vi "active_tracks_functional_global.vi"(4 "StimulusObjectInput":refnum<class "StimulusObject.lvclass">, 6 "Camera Frame In":i32, 7 "Track Index In":i32, 8 "error in":errorcluster, 9 "Operations":T5, 10 "Track Snippets In":T2[](array[typedef]), 11 "Full Worm Track In":T4) -> (0 "error out":errorcluster, 1 "Stimulus Snippets Out":T1[](array[typedef]), 2 "Track Snippets Out":T2[](array[typedef]), 3 "Full Worm Track Out":T4, 5 "Active Track Indecies":i32[](array[numeric]))   [LabVIEW 2019]
uses:
  ActiveTracksFunctionalGlobalOperations.ctl
  WormTrackCluster.ctl
  StimulusObject.lvclass
  TrackTerminationReasonEnum.ctl
  WormTrackSnippetCluster.ctl
  StimulusSnippetCluster.ctl
  CompletedTracksFunctionalGlobalOperations.ctl
  StimulusObject.lvclass/StimulusObject.ctl
  flip_2D_single_array_td.vi
  ParametersGlobal.vi
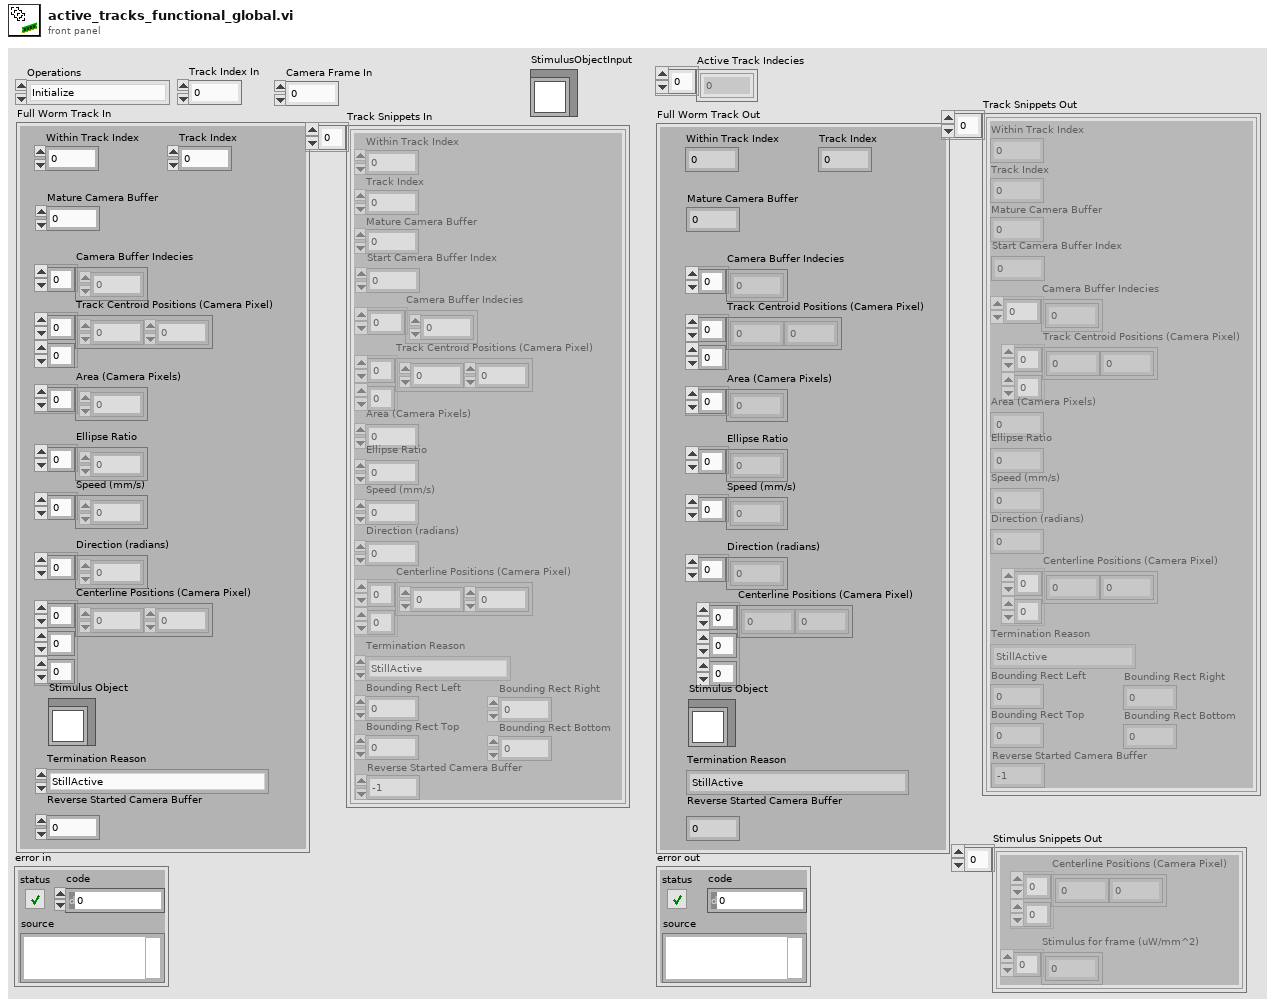
[diagram p1: front panel]
types:
  T1 = typedef "StimulusSnippetCluster.ctl" = cluster{"Centerline Positions (Camera Pixel)":sgl[][], "Stimulus for frame (uW/mm^2)":sgl[]}
  T2 = typedef "WormTrackSnippetCluster.ctl" = cluster{"Track Centroid Positions (Camera Pixel)":sgl[][], "Within Track Index":i32, "Camera Buffer Indecies":i32[], "Area (Camera Pixels)":i32, "Speed (mm/s)":sgl, "Direction (radians)":sgl, "Centerline Positions (Camera Pixel)":sgl[][], "Ellipse Ratio":sgl, "Termination Reason":T3, "Track Index":i32, "Bounding Rect Left":i32, "Bounding Rect Top":i32, "Bounding Rect Right":i32, "Bounding Rect Bottom":i32, "Mature Camera Buffer":i32, "Start Camera Buffer Index":i32, "Reverse Started Camera Buffer":i32}
  T3 = typedef "TrackTerminationReasonEnum.ctl" = enum16{"StillActive", "MaxDisplacement", "NoBlobsLeft", "AreaIncrease", "AreaDecrease", "ExperimentEnded"}
  T4 = typedef "WormTrackCluster.ctl" = cluster{"Track Centroid Positions (Camera Pixel)":sgl[][], "Within Track Index":i32, "Camera Buffer Indecies":i32[], "Area (Camera Pixels)":i32[], "Speed (mm/s)":sgl[], "Direction (radians)":sgl[], "Centerline Positions (Camera Pixel)":sgl[][][], "Ellipse Ratio":sgl[], "Stimulus Object":refnum<class "StimulusObject.lvclass">, "Termination Reason":T3, "Track Index":i32, "Mature Camera Buffer":i32, "Reverse Started Camera Buffer":i32}
  T5 = typedef "ActiveTracksFunctionalGlobalOperations.ctl" = enum16{"Initialize", "ReadFullTrackGivenWormIndex", "WriteFullTrack", "ReadTrackSnippets", "WriteTrackGivenSnippets", "ReadStimulusSnippets", "StartNewTracksGivenSnippets", "EndTracksGivenSnippets", "WriteStimulusObjectGivenWormIndex", "CompleteAllActiveTracks", "ReturnAllActiveTrackIndecies"}
  T6 = typedef "CompletedTracksFunctionalGlobalOperations.ctl" = enum16{"Initialize", "ReturnAllTracks", "ReturnLastIndex", "SaveCompletedTracks", "TrimAndReturnAllTracks"}
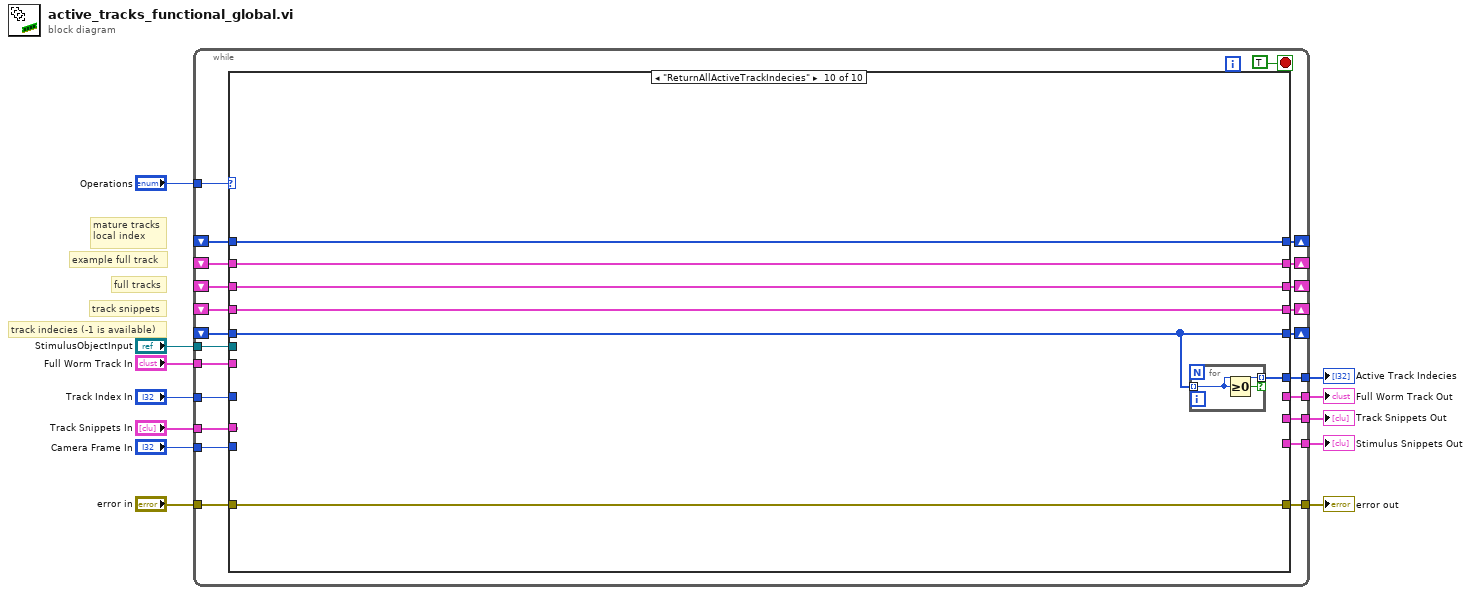
[diagram p0: block diagram]
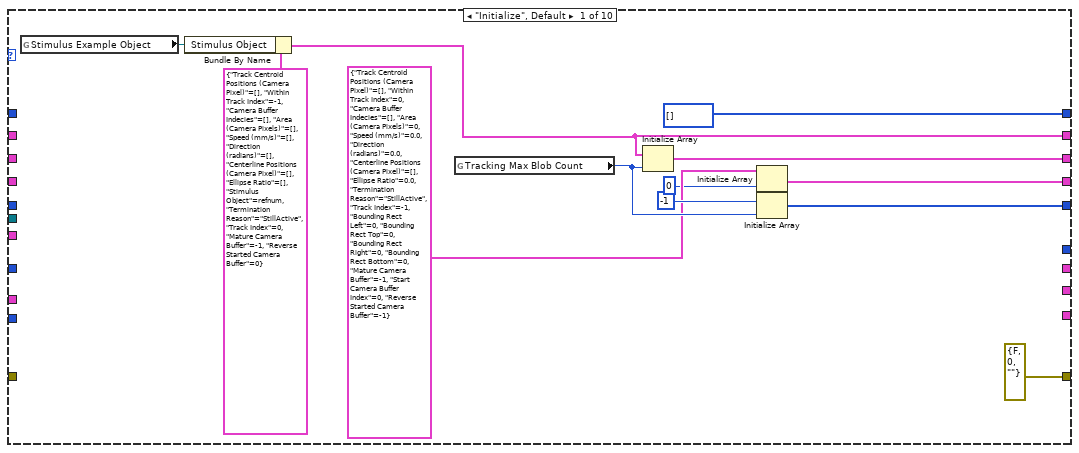
[diagram p2: hidden frame]
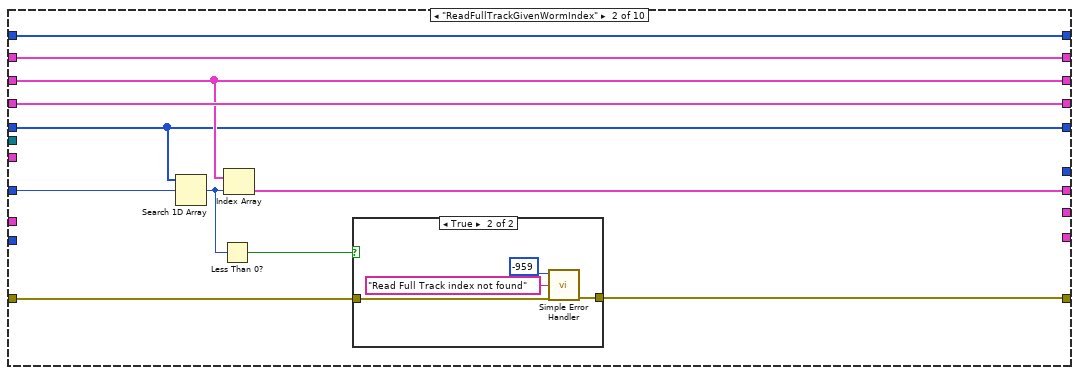
[diagram p3: hidden frame]
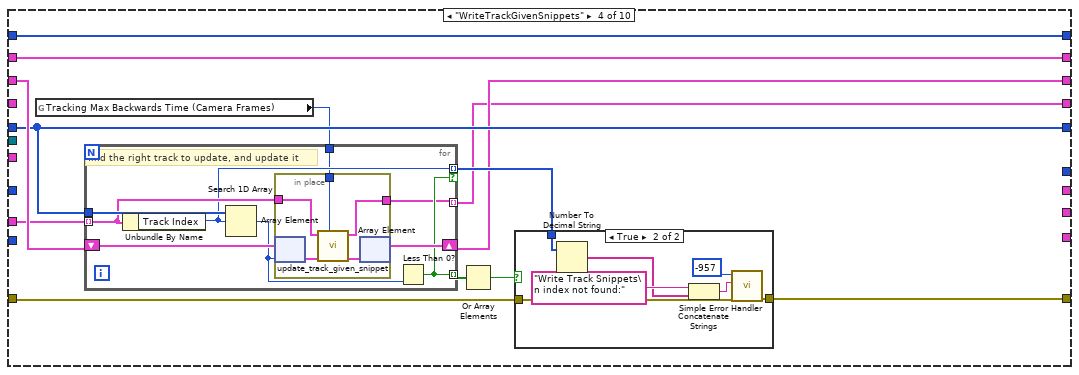
[diagram p6: hidden frame]
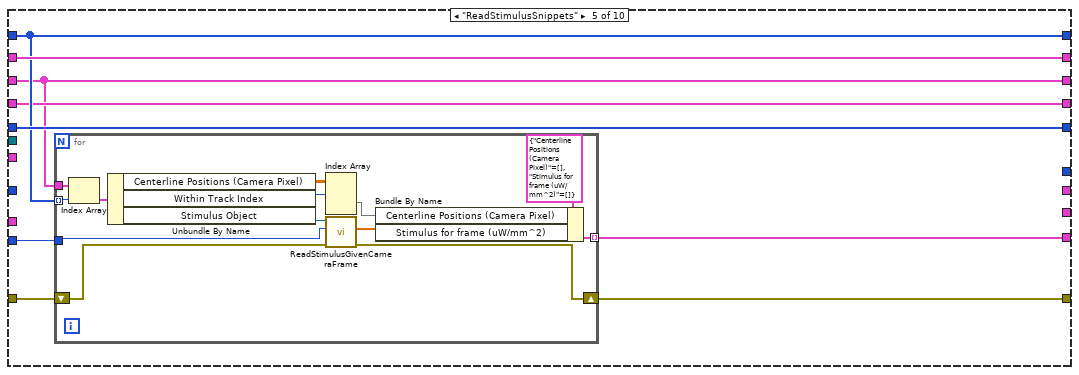
[diagram p8: hidden frame]
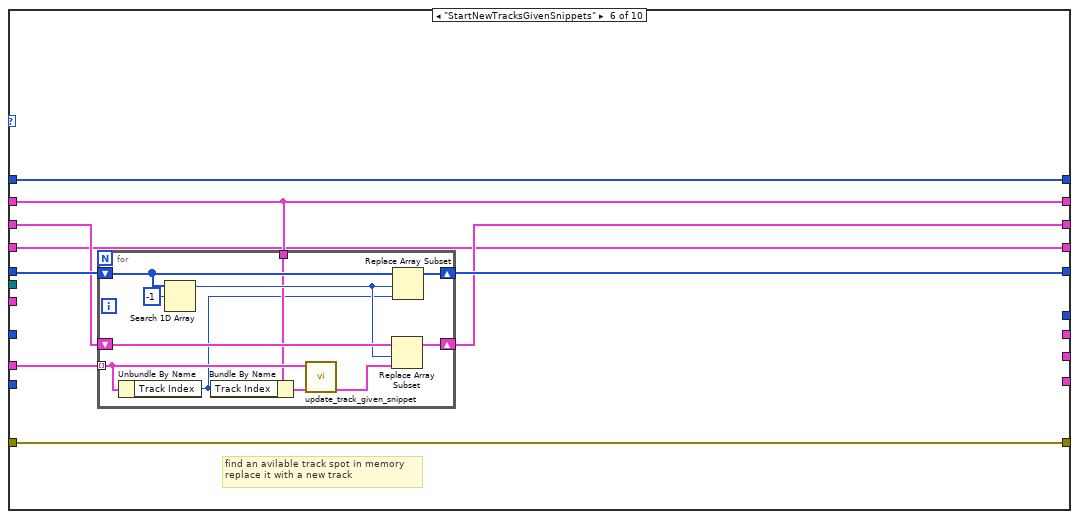
[diagram p9: hidden frame]
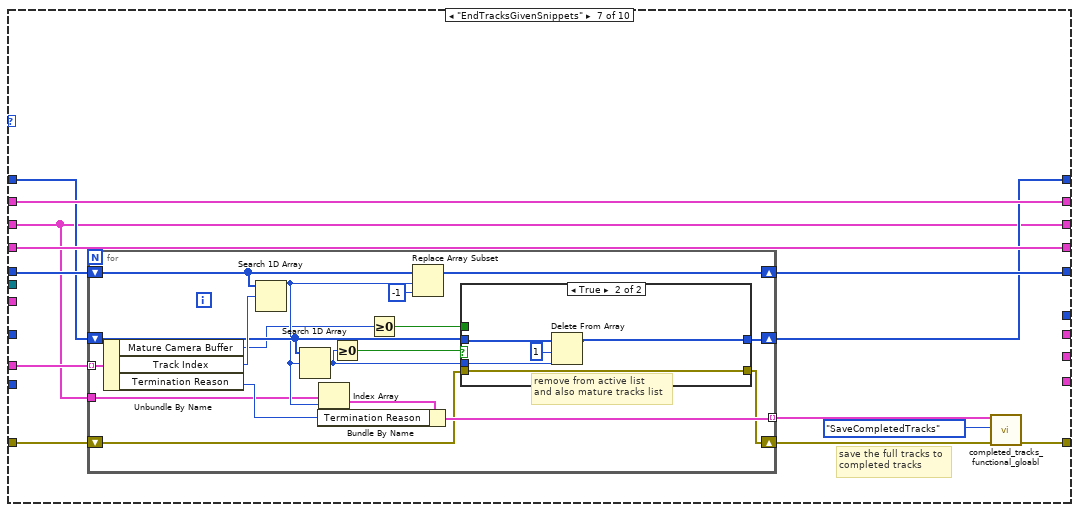
[diagram p10: hidden frame]
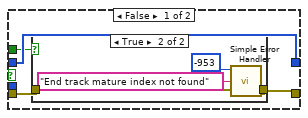
[diagram p11: hidden frame]
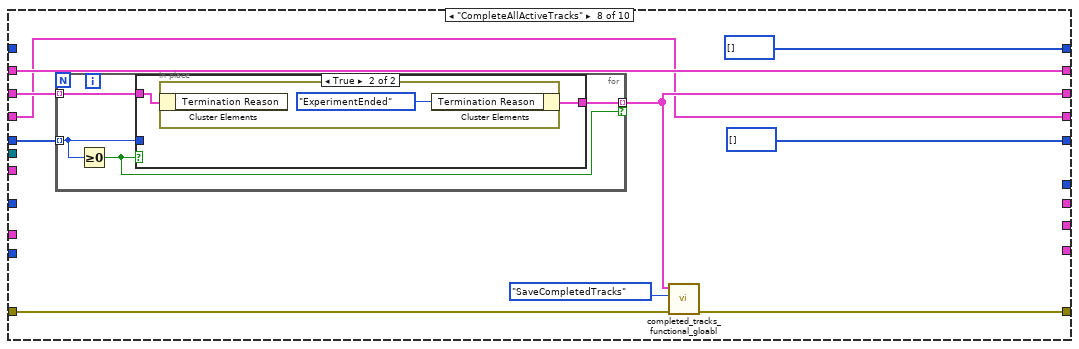
[diagram p13: hidden frame]
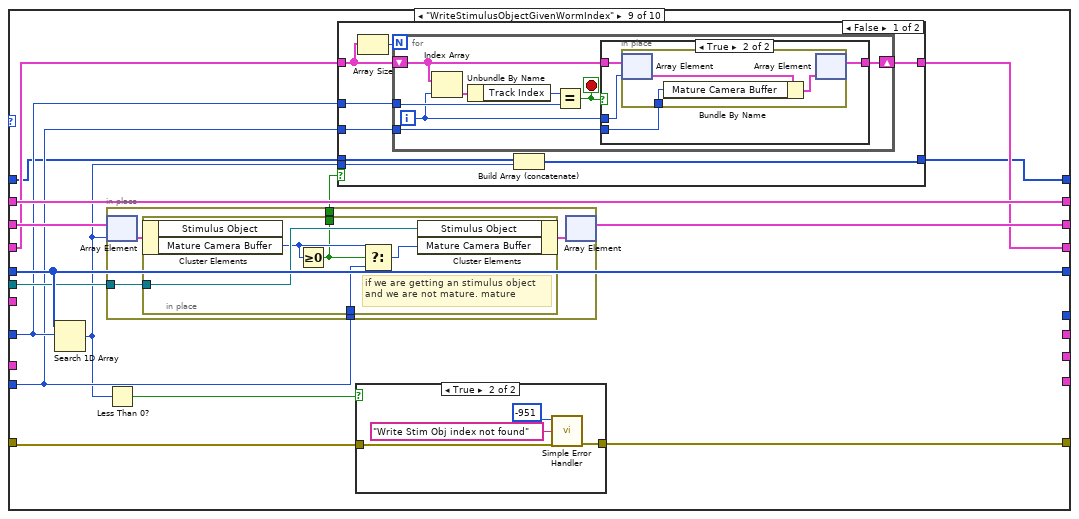
[diagram p15: hidden frame]
diagram:
  # "mature tracks\nlocal index"
  # "example full track"
  # "track indecies (-1 is available)"
  # "track snippets"
  # "full tracks"
  n1 = while {
    shift-right: [w25] -> _
    shift-left: _ -> [w30]
    shift-right: [w32] -> _
    shift-left: _ -> [w29]
    shift-right: [w33] -> _
    shift-left: _ -> [w28]
    shift-right: [w34] -> _
    shift-left: _ -> [w31]
    shift-right: [w27] -> _
    shift-left: _ -> [w26]
    tunnel: "Operations" -> [w24]
    tunnel: "Camera Frame In" -> [w23]
    tunnel: "Track Index In" -> [w22]
    tunnel: "Track Snippets In" -> [w21]
    tunnel: "error in" -> [w20]
    tunnel: [w19] -> w7
    tunnel: [w18] -> w6
    tunnel: [w17] -> w5
    tunnel: [w16] -> w4
    tunnel: "Full Worm Track In" -> [w15]
    tunnel: "StimulusObjectInput" -> [w14]
    tunnel: [w13] -> w1
    stop <- TRUE stop-if-true
    n2 = case shown="\"ReturnAllActiveTrackIndecies\"" w24 {
      tunnel: [w45 w56 w68 w72 w109 w131 w149 w193 w222 w271] -> w25
      tunnel: [w44 w58 w69 w81 w113 w130 w159 w200 w221 w272] -> w34
      tunnel: [w41 w55 w67 w73 w112 w134 w156 i32[] [] w220 w269] -> w33
      tunnel: [w38 w57 w64 w71 w110 w127 w154 w192 w216 w270] -> w32
      tunnel: w31 -> [_ w58 w69 w81 w113 w130 w159 w200 w221 w272]
      tunnel: w30 -> [_ w56 w68 w82 w109 w132 w149 w198 w223 w271]
      tunnel: w29 -> [_ w57 w64 _ w110 w127 w154 w192 w217 w270]
      tunnel: w28 -> [_ w55 w67 w73 w112 w135 w158 w199 w220 w269]
      tunnel: w21 -> [_ _ _ w80 _ w133 w157 _ _ _]
      tunnel: [errorcluster {"status"=FALSE, "code"=0, "source"=""} ("error out") w50 w66 w76 w107 w129 w152 w196 w224 w267] -> w19
      tunnel: w20 -> [_ w51 w66 w77 w108 w129 w148 w197 w225 w267]
      tunnel: [i32[] [] w54 w65 w79 w111 w128 w150 i32[] [] w212 w273] -> w27
      tunnel: w26 -> [_ w54 w65 w79 w111 w128 w151 _ w213 w273]
      tunnel: w22 -> [_ w49 _ _ _ _ _ _ w215 _]
      tunnel: w23 -> [_ _ _ _ w106 _ _ _ w214 _]
      tunnel: [_ w48 _ _ _ _ _ _ _ _] -> w18
      tunnel: [_ _ w64 _ _ _ _ _ _ _] -> w17
      tunnel: [_ _ _ _ w105 _ _ _ _ _] -> w16
      tunnel: w15 -> [_ _ _ _ _ _ _ _ _ _]
      tunnel: w14 -> [_ _ _ _ _ _ _ _ w219 _]
      tunnel: [_ _ _ _ _ _ _ _ _ w268] -> w13
      frame "Initialize", Default {
        n3 = global read "ParametersGlobal.vi" "Stimulus Example Object"() -> (w47:refnum<class "StimulusObject.lvclass">)
        n4 = Bundle By Name(cluster=T4 {"Track Centroid Positions (Camera Pixel)"=[], "Within Track Index"=-1, "Camera Buffer Indecies"=[], "Area (Camera Pixels)"=[], "Speed (mm/s)"=[], "Direction (radians)"=[], "Centerline Positions (Camera Pixel)"=[], "Ellipse Ratio"=[], "Stimulus Object"=refnum, "Termination Reason"=enum."StillActive", "Track Index"=0, "Mature Camera Buffer"=-1, "Reverse Started Camera Buffer"=0} ("Tracks"), "Stimulus Object"=w47) -> (w44:T4)
        n5 = global read "ParametersGlobal.vi" "Tracking Max Blob Count"() -> (w43:i32)
        n6 = Initialize Array(w44, w43) -> (w45:T4[])
        n7 = Initialize Array(T2 {"Track Centroid Positions (Camera Pixel)"=[], "Within Track Index"=0, "Camera Buffer Indecies"=[], "Area (Camera Pixels)"=0, "Speed (mm/s)"=0.0, "Direction (radians)"=0.0, "Centerline Positions (Camera Pixel)"=[], "Ellipse Ratio"=0.0, "Termination Reason"=enum."StillActive", "Track Index"=-1, "Bounding Rect Left"=0, "Bounding Rect Top"=0, "Bounding Rect Right"=0, "Bounding Rect Bottom"=0, "Mature Camera Buffer"=-1, "Start Camera Buffer Index"=0, "Reverse Started Camera Buffer"=-1}, 0 ("dimension size")) -> (w38:T2[])
        n8 = Initialize Array(-1, w43) -> (w41:i32[])
      }
      frame "ReadFullTrackGivenWormIndex" {
        n9 = Search 1D Array(1D array=w55, element=w49) -> (index of element=w53:i32)  [unwired: 1 in]
        n10 = Less Than 0?(x=w53) -> (x < 0?=w52:bool)
        n11 = Index Array(array=w56, index=w53) -> (element=w48:T4)
        n12 = case shown="True" w52 {
          tunnel: w51 -> [w59 w63]
          tunnel: [w59 w62] -> w50
          frame False {
          }
          frame True {
            n13 = call <vilib>:"Simple Error Handler.vi"("error code (no error:0)"=-959, "error source (\" \")"="Read Full Track index not found" ("error source (\" \")"), "error in (no error)"=w63) -> ("error out"=w62:errorcluster)  [unwired: 2 in, 4 out]
          }
        }
      }
      frame "ReadTrackSnippets" {
      }
      frame "WriteTrackGivenSnippets" {
        n14 = global read "ParametersGlobal.vi" "Tracking Max Backwards Time (Camera Frames)"() -> (w70:i32)
        n15 = for {
          tunnel: w80 -> [w97] mode=indexing
          tunnel: w73 -> [w99]
          shift-right: [w96] -> w72
          shift-left: w82 -> [w98]
          tunnel: [w93] -> w78 mode=indexing
          tunnel: [w94] -> w74 mode=indexing if=w93
          tunnel: [w92] -> w71 mode=indexing
          tunnel: w70 -> [w91]
          # "find the right track to update, and update it"
          n16 = Unbundle By Name(w97) -> ("Track Index"=w94:i32)
          n17 = Search 1D Array(1D array=w99, element=w94) -> (index of element=w95:i32)  [unwired: 1 in]
          n18 = in-place {
            in-place-border: w97 -> [w102]
            in-place-border: [w101] -> w92
            in-place-border: w91 -> [w100]
            n19 = in-place-array #1(w98, w95) -> (w104:T4)
            n20 = call "update_track_given_snippet.vi"("Tracking Max Backwards Time (Camera Frames)"=w100, "Input Track"=w104, "Track Snippet In"=w102) -> ("Output Track"=w103:T4, "Track Snippet Out"=w101:T2)  [unwired: 7 in]
            n21 = in-place-array #1(w103) -> (w96:T4[])  [unwired: 1 out]
          }
          n22 = Less Than 0?(x=w95) -> (x < 0?=w93:bool)
        }
        n23 = Or Array Elements(Boolean array=w78) -> (logical OR=w75:bool)
        n24 = case shown="True" w75 {
          tunnel: w77 -> [w83 w90]
          tunnel: [w83 w89] -> w76
          tunnel: w74 -> [_ w87]
          frame False {
          }
          frame True {
            n25 = Number To Decimal String(number=w87) -> (decimal integer string=w84:string[])  [unwired: 1 in]
            n26 = Concatenate Strings("Write Track Snippets\n index not found:" ("error source (\" \")"), w84) -> (w86:string)
            n27 = call <vilib>:"Simple Error Handler.vi"("error code (no error:0)"=-957, "error source (\" \")"=w86, "error in (no error)"=w90) -> ("error out"=w89:errorcluster)  [unwired: 2 in, 4 out]
          }
        }
      }
      frame "ReadStimulusSnippets" {
        n28 = for {
          tunnel: w111 -> [w125] mode=indexing
          tunnel: w109 -> [w126]
          tunnel: [w117] -> w105 mode=indexing
          shift-right: [w115] -> w107
          shift-left: w108 -> [w116]
          tunnel: w106 -> [w114]
          n29 = Index Array(array=w126, index=w125) -> (element=w124:T4)
          n30 = Unbundle By Name(w124) -> ("Centerline Positions (Camera Pixel)"=w123:sgl[][][], "Within Track Index"=w122:i32, "Stimulus Object"=w121:refnum<class "StimulusObject.lvclass">)
          n31 = Index Array(array=w123, index (dim 0)=w122) -> (element=w118:sgl[][])  [unwired: 2 in]
          n32 = call "ReadStimulusGivenCameraFrame.vi"("error in (no error)"=w116, "CameraFrame"=w114, "StimulusObject in"=w121) -> ("error out"=w115:errorcluster, "StimulusForFrame"=w119:sgl[])  [unwired: 6 in, 1 out]
          n33 = Bundle By Name(cluster=T1 {"Centerline Positions (Camera Pixel)"=[], "Stimulus for frame (uW/mm^2)"=[]}, "Centerline Positions (Camera Pixel)"=w118, "Stimulus for frame (uW/mm^2)"=w119) -> (w117:T1)
        }
      }
      frame "StartNewTracksGivenSnippets" {
        # "find an avilable track spot in memory\nreplace it with a new track"
        n34 = for {
          tunnel: w133 -> [w145] mode=indexing
          shift-right: [w144] -> w131
          shift-left: w132 -> [w146]
          shift-right: [w140] -> w134
          shift-left: w135 -> [w142]
          tunnel: w130 -> [w139]
          n35 = Unbundle By Name(w145) -> ("Track Index"=w136:i32)
          n36 = Search 1D Array(1D array=w142, element=-1) -> (index of element=w141:i32)  [unwired: 1 in]
          n37 = Bundle By Name(cluster=w139, "Track Index"=w136) -> (w137:T4)
          n38 = call "update_track_given_snippet.vi"("Input Track"=w137, "Track Snippet In"=w145) -> ("Output Track"=w138:T4)  [unwired: 8 in, 1 out]
          n39 = Replace Array Subset(array=w146, new element=w138, index=w141) -> (w144:T4[])
          n40 = Replace Array Subset(array=w142, new element=w136, index=w141) -> (w140:i32[])
        }
      }
      frame "EndTracksGivenSnippets" {
        # "save the full tracks to\ncompleted tracks"
        n41 = for {
          shift-right: [w175] -> w156
          shift-left: w158 -> [w176]
          tunnel: w157 -> [w177] mode=indexing
          tunnel: [w169] -> w153 mode=indexing
          shift-right: [w172] -> w150
          shift-left: w151 -> [w167]
          tunnel: w149 -> [w164]
          shift-right: [w162] -> w147
          shift-left: w148 -> [w163]
          # "remove from active list\nand also mature tracks list"
          n42 = Unbundle By Name(w177) -> ("Mature Camera Buffer"=w161:i32, "Track Index"=w174:i32, "Termination Reason"=w168:T3)
          n43 = Search 1D Array(1D array=w176, element=w174) -> (index of element=w165:i32)  [unwired: 1 in]
          n44 = Search 1D Array(1D array=w167, element=w165) -> (index of element=w166:i32)  [unwired: 1 in]
          n45 = Index Array(array=w164, index=w165) -> (element=w170:T4)
          n46 = Bundle By Name(cluster=w170, "Termination Reason"=w168) -> (w169:T4)
          n47 = Greater Or Equal To 0?(x=w166) -> (x >= 0?=w173:bool)
          n48 = Greater Or Equal To 0?(x=w161) -> (x >= 0?=w160:bool)
          n49 = Replace Array Subset(array=w176, new element=-1 ("element"), index=w165) -> (w175:i32[])
          n50 = case shown="True" w173 {
            tunnel: w166 -> [_ w191]
            tunnel: w167 -> [w180 w189]
            tunnel: [w180 w188] -> w172
            tunnel: w163 -> [w179 w187]
            tunnel: [w181 w187] -> w162
            tunnel: w160 -> [w178 _]
            frame False {
              n51 = case shown="True" w178 {
                tunnel: [w182 w184] -> w181
                tunnel: w179 -> [w182 w183]
                frame False {
                }
                frame True {
                  n52 = call <vilib>:"Simple Error Handler.vi"("error code (no error:0)"=-953, "error source (\" \")"="End track mature index not found" ("error source (\" \")"), "error in (no error)"=w183) -> ("error out"=w184:errorcluster)  [unwired: 2 in, 4 out]
                }
              }
            }
            frame True {
              n53 = Delete From Array(array=w189, length=1, index=w191) -> (array with subset deleted=w188:i32[])  [unwired: 1 out]
            }
          }
        }
        n54 = call "completed_tracks_functional_gloabl.vi"("error in (no error)"=w147, 10:CompletedTracksFunctionalGlobalOperations."SaveCompletedTracks", "CompletedTracksToSave"=w153) -> ("error out"=w152:errorcluster)  [unwired: 5 in, 3 out]
      }
      frame "CompleteAllActiveTracks" {
        n55 = for {
          tunnel: w199 -> [w205] mode=indexing
          tunnel: w198 -> [w204] mode=indexing
          tunnel: [w203] -> w193 mode=indexing if=w202
          n56 = Greater Or Equal To 0?(x=w205) -> (x >= 0?=w202:bool)
          n57 = case shown="True" w202 {
            tunnel: w205 -> [_ _]
            tunnel: w204 -> [w206 w208]
            tunnel: [w206 w207] -> w203
            frame False {
            }
            frame True {
              n58 = in-place {
                n59 = in-place-cluster #2(w208) -> ()  [unwired: 1 out]
                n60 = in-place-cluster #2("Termination Reason"=TrackTerminationReasonEnum."ExperimentEnded") -> (w207:T4)
              }
            }
          }
        }
        n61 = call "completed_tracks_functional_gloabl.vi"("error in (no error)"=w197, 10:CompletedTracksFunctionalGlobalOperations."SaveCompletedTracks", "CompletedTracksToSave"=w193) -> ("error out"=w196:errorcluster)  [unwired: 5 in, 3 out]
      }
      frame "WriteStimulusObjectGivenWormIndex" {
        n62 = Search 1D Array(1D array=w220, element=w215) -> (index of element=w211:i32)  [unwired: 1 in]
        n63 = in-place {
          in-place-border: w219 -> [w255]
          in-place-border: w214 -> [w253]
          in-place-border: [w252] -> w218
          n64 = in-place-array #3(w223, w211) -> (w256:T4)
          n65 = in-place {
            in-place-border: w255 -> [w261]
            in-place-border: w253 -> [w258]
            in-place-border: [w257] -> w252
            # "if we are getting an stimulus object\nand we are not mature. mature"
            n66 = in-place-cluster #4(w256) -> ("Mature Camera Buffer"=w260:i32)  [unwired: 1 out]
            n67 = Greater Or Equal To 0?(x=w260) -> (x >= 0?=w257:bool)
            n68 = Select(t=w260, s=w257, f=w258) -> (s? t:f=w259:i32)
            n69 = in-place-cluster #4("Stimulus Object"=w261, "Mature Camera Buffer"=w259) -> (w254:T4)
          }
          n70 = in-place-array #3(w254) -> (w222:T4[])  [unwired: 1 out]
        }
        n71 = Less Than 0?(x=w211) -> (x < 0?=w210:bool)
        n72 = case shown="False" w218 {
          tunnel: w213 -> [w233 w251]
          tunnel: [w232 w251] -> w212
          tunnel: w215 -> [w231 _]
          tunnel: w217 -> [w227 w250]
          tunnel: [w228 w250] -> w216
          tunnel: w214 -> [w230 _]
          tunnel: w211 -> [w229 _]
          frame False {
            n73 = Array Size(array=w227) -> (size(s)=w226:i32)
            n74 = for {
              N: w226 -> [_]
              tunnel: w231 -> [w240]
              tunnel: w230 -> [w239]
              shift-right: [w235] -> w228
              shift-left: w227 -> [w237]
              i -> [w234]
              stop <- w238 stop-if-true
              n75 = Index Array(array=w237, index=w234) -> (element=w236:T2)
              n76 = Unbundle By Name(w236) -> ("Track Index"=w241:i32)
              n77 = Equal?(x=w241, y=w240) -> (x = y?=w238:bool)
              n78 = case shown="True" w238 {
                tunnel: w237 -> [w242 w246]
                tunnel: [w242 w243] -> w235
                tunnel: w239 -> [_ w244]
                tunnel: w234 -> [_ w245]
                frame False {
                }
                frame True {
                  n79 = in-place {
                    in-place-border: w244 -> [w249]
                    n80 = in-place-array #5(w246, w245) -> (w248:T2)
                    n81 = Bundle By Name(cluster=w248, "Mature Camera Buffer"=w249) -> (w247:T2)
                    n82 = in-place-array #5(w247) -> (w243:T2[])  [unwired: 1 out]
                  }
                }
              }
            }
            n83 = Build Array (concatenate)(w233, w229) -> (w232:i32[])
          }
          frame True {
          }
        }
        n84 = case shown="True" w210 {
          tunnel: w225 -> [w262 w266]
          tunnel: [w262 w265] -> w224
          frame False {
          }
          frame True {
            n85 = call <vilib>:"Simple Error Handler.vi"("error code (no error:0)"=-951, "error source (\" \")"="Write Stim Obj index not found" ("error source (\" \")"), "error in (no error)"=w266) -> ("error out"=w265:errorcluster)  [unwired: 2 in, 4 out]
          }
        }
      }
      frame "ReturnAllActiveTrackIndecies" {
        n86 = for {
          tunnel: w269 -> [w275] mode=indexing
          tunnel: [w275] -> w268 mode=indexing if=w274
          n87 = Greater Or Equal To 0?(x=w275) -> (x >= 0?=w274:bool)
        }
      }
    }
  }
  "error out" <- w7
  "Full Worm Track Out" <- w6
  "Track Snippets Out" <- w5
  "Stimulus Snippets Out" <- w4
  "Active Track Indecies" <- w1
